vi "PIcontroller.vi"(1 "min":fxp<+/-,15,-7>=-0.003301858901977539 format="%#_50g", 2 "max":fxp<+,15,-8>=0.00330197811126709 format="%#_51g", 3 "KiTs":fxp<+,11,-22>=1.25030055642128e-07 format="%#_61g", 4 "Kp":fxp<+/-,32,-4>, 5 "e[k]":fxp<+/-,32,-4>, 6 "reset":bool) -> (0 "u[k]":fxp<+/-,47,-5> format="%.67g")   [LabVIEW 2020]
uses:
  <vilib>/rvi/Emulation/niFpgaSctlEmulationGetInTimedLoop.vi
  <vilib>/rvi/Emulation/niFpgaProcessEmulError.vi
panel:
  in  "sat":fxp<+/-,2,2>
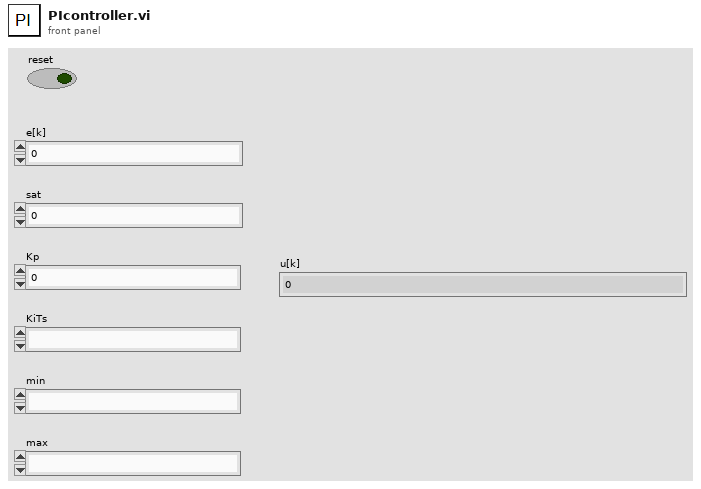
[diagram p1: front panel]
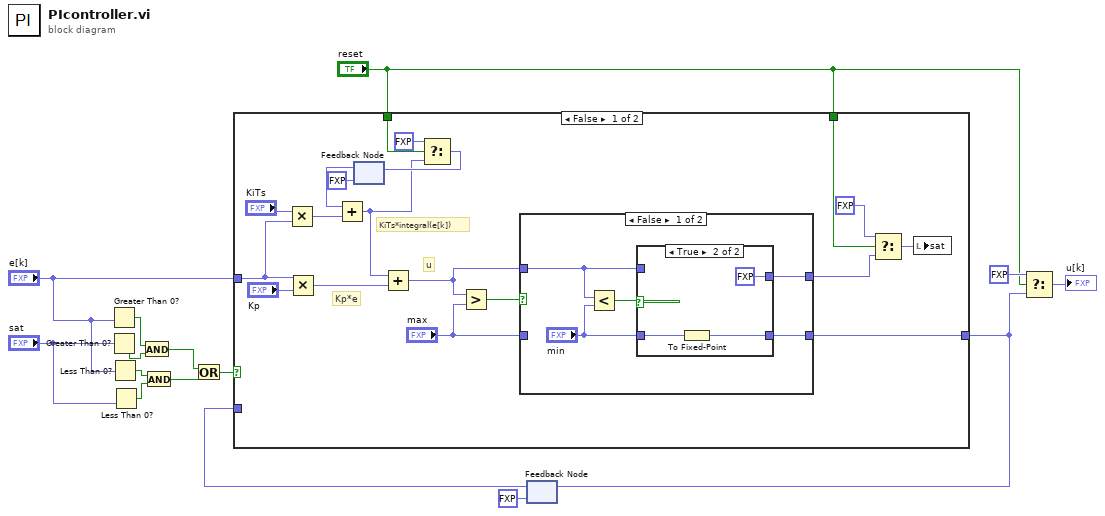
[diagram p0: block diagram]
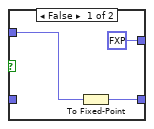
[diagram p2: hidden frame]
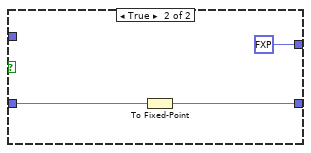
[diagram p3: hidden frame]
diagram:
  n1 = Greater Than 0?(x="e[k]") -> (x > 0?=w12:bool)
  n2 = Greater Than 0?(x="sat") -> (x > 0?=w11:bool)
  n3 = Less Than 0?(x="e[k]") -> (x < 0?=w10:bool)
  n4 = Less Than 0?(x="sat") -> (x < 0?=w9:bool)
  n5 = And(x=w12, y=w11) -> (x .and. y?=w14:bool)
  n6 = And(x=w10, y=w9) -> (x .and. y?=w13:bool)
  n7 = Or(x=w14, y=w13) -> (x .or. y?=w15:bool)
  n8 = feedback #1(fxp<+/-,47,-5> 0.0 ("upper limit")) -> (w6:fxp<+/-,47,-5>)
  n9 = case shown="False" w15 {
    tunnel: "e[k]" -> [w33 _]
    tunnel: [w30 w49] -> w3
    tunnel: w6 -> [_ w49]
    tunnel: "reset" -> [w17 _]
    tunnel: "reset" -> [w16 _]
    frame False {
      # "u"
      # "Kp*e"
      # "KiTs*integral(e[k])"
      n10 = Multiply(x="KiTs", y=w33) -> (x*y=w26:fxp<+/-,32,-27>)
      n11 = Multiply(x=w33, y="Kp") -> (x*y=w28:fxp<+/-,42,-10>)
      n12 = feedback #2(fxp<+,44,-6> 0.0) -> (w27:fxp<+/-,45,-5>)
      n13 = Add(x=w27, y=w26) -> (x+y=w18:fxp<+/-,44,-6>)
      n14 = Add(x=w18, y=w28) -> (x+y=w31:fxp<+/-,47,-5>)
      n15 = Select(t=fxp<+/-,44,-6> 0.0, s=w17, f=w18) -> (s? t:f=w20:fxp<+/-,44,-6>)
      n16 = feedback-in #2(w20) -> ()
      n17 = Greater?(x=w31, y="max") -> (0:w32:bool)
      n18 = case shown="False" w32 {
        tunnel: w31 -> [w35 _]
        tunnel: [w38 w46] -> w30
        tunnel: "max" -> [_ w47]
        tunnel: [w37 fxp<+/-,2,2> 1.0 ("sat")] -> w22
        frame False {
          n19 = Less?(x=w35, y="min") -> (x < y?=w39:bool)
          n20 = case shown="True" w39 {
            tunnel: [w40 w43] -> w38
            tunnel: w35 -> [w41 _]
            tunnel: "min" -> [_ w44]
            tunnel: [fxp<+/-,2,2> 0.0 ("sat") fxp<+/-,1,1> -1.0 ("sat")] -> w37
            frame False {
              n21 = To Fixed-Point(number=w41) -> (fixed-point=w40:fxp<+/-,47,-5>)  [unwired: 1 in]
            }
            frame True {
              n22 = To Fixed-Point(number=w44) -> (fixed-point=w43:fxp<+/-,47,-5>)  [unwired: 1 in]
            }
          }
        }
        frame True {
          n23 = To Fixed-Point(number=w47) -> (fixed-point=w46:fxp<+/-,47,-5>)  [unwired: 1 in]
        }
      }
      n24 = Select(t=fxp<+/-,2,2> 0.0, s=w16, f=w22) -> (s? t:f=w24:fxp<+/-,2,2>)
      n25 = local write "sat"(w24) -> ()
    }
    frame True {
    }
  }
  n26 = feedback-in #1(w3) -> ()
  n27 = Select(t=fxp<+/-,47,-5> 0.0, s="reset", f=w3) -> (s? t:f=→"u[k]":fxp<+/-,47,-5>)
